vi "Position Move.vi"(10 "Target":i32=127, 11 "Spliter":refnum<vi>) -> ()   [LabVIEW 2020]
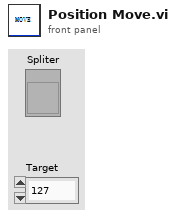
[diagram p1: front panel]
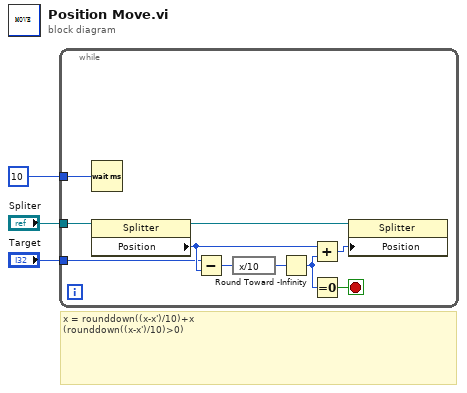
[diagram p0: block diagram]
diagram:
  # "x = rounddown((x-x')/10)+x\n(rounddown((x-x')/10)>0)"
  n1 = while {
    tunnel: "Spliter" -> [w13]
    tunnel: "Target" -> [w7]
    tunnel: u32 10 ("Delay(ms)") -> [w4]
    stop <- w5 stop-if-true
    n2 = Wait (ms)(milliseconds to wait=w4) -> ()  [unwired: 1 out]
    n3 = property class="Splitter"(reference=w13) -> (reference out=w12:refnum<vi>, "Position"=w9:i32)  [unwired: 1 in, 1 out]
    n4 = Subtract(x=w7, y=w9) -> (x-y=w11:i32)
    n5 = expression code="x/10"(w11) -> (w10:i32)
    n6 = Round Toward -Infinity(1:w10) -> (0:w6:i32)
    n7 = Add(x=w9, y=w6) -> (x+y=w8:i32)
    n8 = Equal To 0?(x=w6) -> (x = 0?=w5:bool)
    n9 = property class="Splitter"(reference=w12, "Position"=w8) -> ()  [unwired: 1 in, 2 out]
  }
